vi "SpecAn Configure AMPM.vi"(0 "RFmx Handle In":refnum<k21>, 1 "Selector String":string, 5 "RFmx SpecAn AMPM Configuration":T1={"Measurement Interval (s)"=0.0001, "DUT Average Input Power (dBm)"=-20.0, "Signal Type"=0, "Averaging Enabled"=0, "Averaging Count"=10, "Reference Waveform"={"Name"="Wfm", "Data"=refnum, "Signal Bandwidth (Hz)"=0.0, "PAPR (dB)"=0.0, "Burst Length (s)"=0.0, "Sample Rate"=0.0, "Burst Start Locations"=[], "Burst Stop Locations"=[], "Idle Duration Present?"=FALSE, "Runtime Scaling"=0.0, "Script"=""}} {"Reference Waveform"."Runtime Scaling" format="%#_6p"; "Reference Waveform"."Sample Rate" format="%#_6p"; "Reference Waveform"."Burst Length (s)" format="%#_6p"; "Reference Waveform"."PAPR (dB)" format="%.2f"; "Reference Waveform"."Signal Bandwidth (Hz)" format="%#_6p"; "Averaging Enabled" items=["False", "True"]; "Signal Type" items=["Modulated", "Tones"]; "DUT Average Input Power (dBm)" format="%.2f"; "Measurement Interval (s)" format="%.2p"}, 11 "error in (no error)":errorcluster) -> (4 "RFmx Handle Out":refnum<k21>, 15 "error out":errorcluster)   [LabVIEW 2019, in "RFmxSpecAn.lvlib"]
doc: "Configures common settings for the AMPM measurement and selects the measurement."
uses:
  RFmxSpecAn.lvlib
  Typedefs/SpecAn AMPM Configuration.ctl
  Common/Waveform.ctl
  <vilib>/RFmx/SpecAn/mx/RFmxSpecAn.llb/RFmxSpecAn Select Measurement (Single).vi
  Common/Common.lvlib
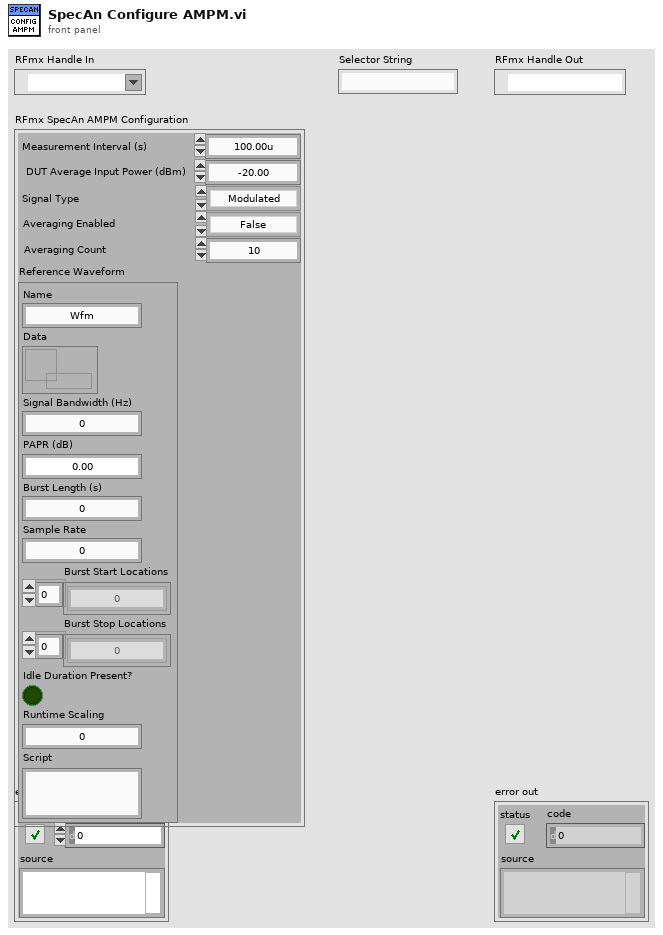
[diagram p1: front panel]
types:
  T1 = typedef "RFmxSpecAn.lvlib/SpecAn AMPM Configuration.ctl" = cluster{"Measurement Interval (s)":dbl, "DUT Average Input Power (dBm)":dbl, "Signal Type":i32, "Averaging Enabled":i32, "Averaging Count":i32, "Reference Waveform":T2}
  T2 = typedef "Common.lvlib/Waveform.ctl" = cluster{"Name":string, "Data":refnum<data-value>, "Signal Bandwidth (Hz)":dbl, "PAPR (dB)":dbl, "Burst Length (s)":dbl, "Sample Rate":dbl, "Burst Start Locations":i32[], "Burst Stop Locations":i32[], "Idle Duration Present?":bool, "Runtime Scaling":dbl, "Script":string}
  T3 = enum16{"ACP", "CCDF", "CHP", "FCnt", "Harmonics", "OBW", "SEM", "Spectrum", "Spur", "TXP", "AMPM", "DPD", "IQ", "IM", "NF", "PhaseNoise", "PAVT"}
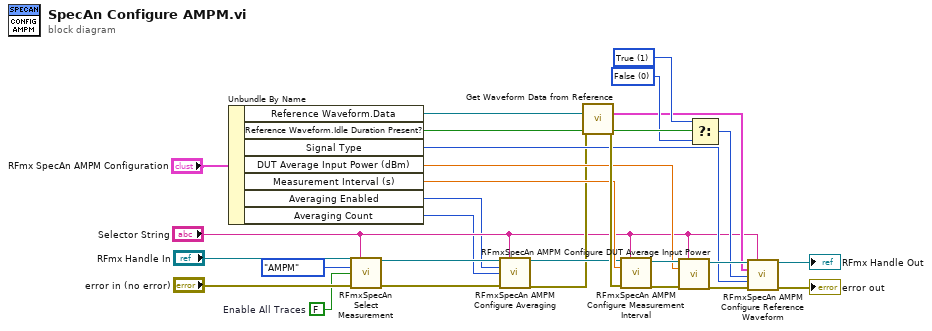
[diagram p0: block diagram]
diagram:
  w8 = FALSE  # Enable All Traces
  w15 = 0 items=["False", "True"] ("Idle Duration Present")
  w18 = 1 items=["False", "True"] ("Idle Duration Present")
  n1 = Unbundle By Name("RFmx SpecAn AMPM Configuration") -> ("Reference Waveform.Data"=w24:refnum<data-value>, "Reference Waveform.Idle Duration Present?"=w16:bool, "Signal Type"=w19:i32, "DUT Average Input Power (dBm)"=w14:dbl, "Measurement Interval (s)"=w13:dbl, "Averaging Enabled"=w2:i32, "Averaging Count"=w1:i32)
  n2 = call-poly <vilib>:"RFmxSpecAn Select Measurement.vi"("Instrument Handle In"="RFmx Handle In", "Selector String"="Selector String", "Measurement"=T3."AMPM", "Enable All Traces"=w8, "error in (no error)"="error in (no error)") -> ("Instrument Handle Out"=w7:refnum<k21>, "error out"=w5:errorcluster)  [unwired: 9 in]
  n3 = call <vilib>:"RFmxSpecAn AMPM Configure Averaging.vi"("Instrument Handle In"=w7, "Selector String"="Selector String", "Averaging Enabled"=w2, "Averaging Count"=w1, "error in (no error)"=w5) -> ("Instrument Handle Out"=w6:refnum<k21>, "error out"=w4:errorcluster)  [unwired: 9 in]
  n4 = call "Get Waveform Data from Reference.vi"("Waveform Data Reference"=w24, "error in (no error)"=w4) -> ("Waveform Data"=w11:cluster{"t0":dbl, "dt":dbl, "y":csg[]}, "error out"=w25:errorcluster)  [unwired: 12 in]
  n5 = call <vilib>:"RFmxSpecAn AMPM Configure Measurement Interval.vi"("Instrument Handle In"=w6, "Selector String"="Selector String", "Measurement Interval (s)"=w13, "error in (no error)"=w25) -> ("Instrument Handle Out"=w23:refnum<k21>, "error out"=w28:errorcluster)  [unwired: 10 in]
  n6 = call <vilib>:"RFmxSpecAn AMPM Configure DUT Average Input Power.vi"("Instrument Handle In"=w23, "Selector String"="Selector String", "DUT Average Input Power (dBm)"=w14, "error in (no error)"=w28) -> ("Instrument Handle Out"=w22:refnum<k21>, "error out"=w27:errorcluster)  [unwired: 10 in]
  n7 = Select(t=w18, s=w16, f=w15) -> (s? t:f=w17:i32)
  n8 = call <vilib>:"RFmxSpecAn AMPM Configure Reference Waveform.vi"("Instrument Handle In"=w22, "Selector String"="Selector String", "Reference Waveform"=w11, "Idle Duration Present"=w17, "Signal Type"=w19, "error in (no error)"=w27) -> ("Instrument Handle Out"=→"RFmx Handle Out":refnum<k21>, "error out"=→"error out":errorcluster)  [unwired: 8 in]
